vi "Check Underflow Warning.vi"(1 "error in(no error)":errorcluster caption="错误输入（无错误）") -> (0 "Module Underflow":bool caption="模块下溢")   [LabVIEW 2013]
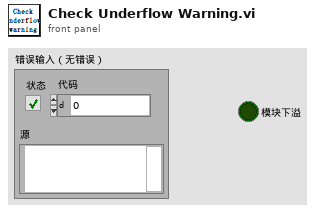
[diagram p1: front panel]
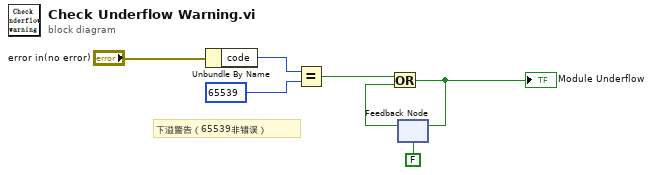
[diagram p0: block diagram]
diagram:
  # "下溢警告（65539非错误）"
  n1 = Unbundle By Name("error in(no error)") -> ("code"=w3:i32)
  n2 = Equal?(x=w3, y=65539) -> (x = y?=w6:bool)
  n3 = feedback #1 ("Latch")(FALSE) -> (w4:bool)
  n4 = Or(x=w6, y=w4) -> (x .or. y?=w1:bool)
  "Module Underflow" <- w1
  n5 = feedback-in #1(w1) -> ()
